vi "(SubVI) Slowly Go to Target PosiitonPI_YCC.vi"(4 "scan rate  (um/s)":dbl=2.0 format="%.3f", 5 "axis":u32=1, 6 "Target position (um)":dbl) -> (1 "step size (nm)":dbl, 2 "Now position (um)":dbl, 3 "True rate?":bool)   [LabVIEW 2014]
panel:
  out "traveling time (s)":dbl
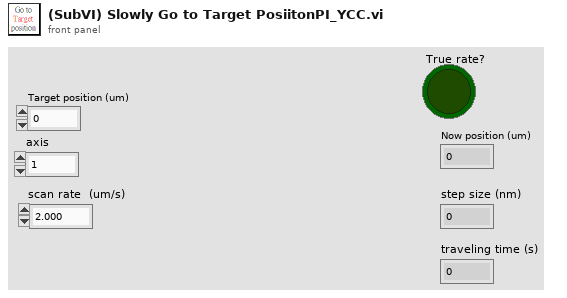
[diagram p1: front panel]
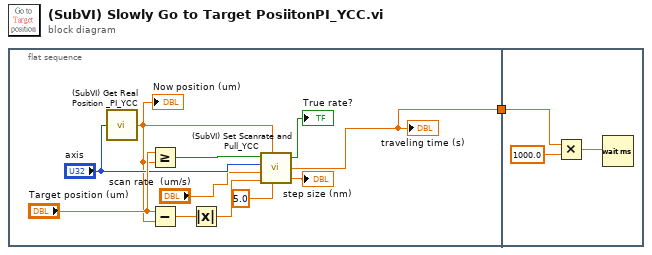
[diagram p0: block diagram]
diagram:
  n1 = flat-sequence {
    tunnel: [w2] -> w1
    tunnel: w1 -> [w13]
    frame #0 {
      n2 = call "(SubVI) Get Real Position _PI_YCC.vi"("Axis"="axis") -> ("Real Current Commanded position (um)"=w4:dbl)  [unwired: 4 in]
      "Now position (um)" <- w4
      n3 = Greater Or Equal?(x="Target position (um)", y=w4) -> (x >= y?=w12:bool)
      n4 = Subtract(x="Target position (um)", y=w4) -> (x-y=w10:dbl)
      n5 = Absolute Value(x=w10) -> (abs(x)=w9:dbl)
      n6 = call "(SubVI) Set Scanrate and Pull_YCC.vi"("toward+ ?\nT=+, F=-"=w12, "Start From  (um)"=w4, "axis"="axis", "scan rate  (um/s)"="scan rate  (um/s)", "waiting time per point (ms)\nrange from 5ms to 0.167 ms"=5.0 ("waiting time per point (ms)\nrange from 5ms to 0.167 ms"), "range  (um)"=w9) -> ("True rate?"=→"True rate?":bool, "traveling time (s)"=w2:dbl, "step size (nm)"=→"step size (nm)":dbl)
      "traveling time (s)" <- w2
    }
    frame #1 {
      n7 = Multiply(x=w13, y=1000.0) -> (x*y=w15:dbl)
      n8 = Wait (ms)(milliseconds to wait=w15) -> ()  [unwired: 1 out]
    }
  }
